vi "Writer.vi"(8 "error in (no error)":errorcluster, 10 "Write Buffer (\"\")":string, 11 "VISA resource name":refnum<visa-resource-name>) -> (0 "error out":errorcluster, 1 "return count":u32, 3 "VISA resource name out":refnum<visa-resource-name>)   [LabVIEW 2013]
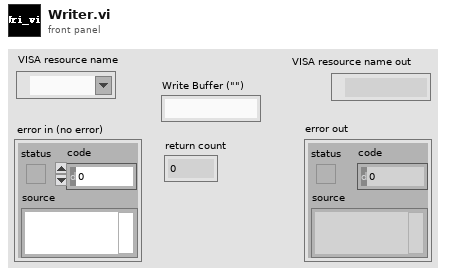
[diagram p1: front panel]
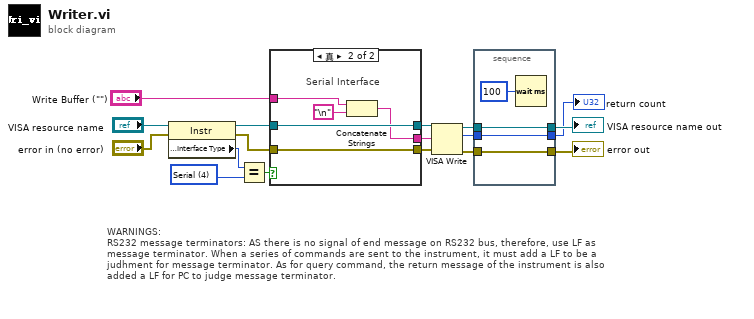
[diagram p0: block diagram]
diagram:
  w14 = u16 4 items=["GPIB"=1, "VXI"=2, "GPIB-VXI"=3, "Serial"=4, "PXI"=5] ("Interface Information:Interface Type")
  # "WARNINGS: \nRS232 message terminators: AS there is no signal of end message on RS232 bus, therefore, use LF as \nmessage terminator. When a series of commands are sent to the instrument, it must add a LF to be a\njudhment for message terminator. As for query command, the return message of the instrument is also\nadded a LF for PC to judge message terminator."
  n1 = property class="Instr"(reference="VISA resource name", error in="error in (no error)") -> (reference out=w15:refnum<visa-resource-name>, error out=w17:errorcluster, "Interface Information:Interface Type"=w13:u16)
  n2 = Equal?(x=w13, y=w14) -> (x = y?=w16:bool)
  n3 = case shown="真" w16 {
    tunnel: w17 -> [w20 w24]
    tunnel: w15 -> [w19 w25]
    tunnel: [w19 w25] -> w8
    tunnel: [w20 w24] -> w9
    tunnel: [w18 w23] -> w7
    tunnel: "Write Buffer (\"\")" -> [w18 w22]
    frame False {
      # "Other Interface"
    }
    frame True {
      # "Serial Interface"
      n4 = Concatenate Strings(w22, "\n") -> (w23:string)
    }
  }
  n5 = VISA Write(VISA resource name=w8, write buffer=w7, error in (no error)=w9) -> (VISA resource name out=w6:refnum<visa-resource-name>, return count=w2:u32, error out=w4:errorcluster)
  n6 = stacked-sequence {
    tunnel: w6 -> [w29]
    tunnel: [w29] -> w5
    tunnel: w4 -> [w28]
    tunnel: [w28] -> w3
    tunnel: w2 -> [w27]
    tunnel: [w27] -> w1
    frame #0 {
      n7 = Wait (ms)(milliseconds to wait=u32 100) -> ()  [unwired: 1 out]
    }
  }
  "error out" <- w3
  "VISA resource name out" <- w5
  "return count" <- w1
